vi "PS Control.vi"() -> ()   [LabVIEW 2025]
doc: "Author: Scott Hannahs <sth@magnet.fsu.edu>\n\nThis software is licensed for use under the “MIT License\"\nCopyright (c) 2025 Scott Hannahs, sth@sth@magnet.sthnet.net\n\nPermission is hereby granted, free of charge, to any person obtaining a copy of this software and associated documentation files (the \"Software\"), to deal in the Software without restriction, including without limitation the rights to use, copy, modify, merge, publish, distribute, sublicense, and/or sell copies of the Software, and to permit persons to whom the Software is furnished to do so, subject to the following conditions: The above copyright notice and this permission notice shall be included in all copies or substantial portions of the Software.\n\nTHE SOFTWARE IS PROVIDED \"AS IS\", WITHOUT WARRANTY OF ANY KIND, EXPRESS OR IMPLIED, INCLUDING BUT NOT LIMITED TO THE WARRANTIES OF MERCHANTABILITY, FITNESS FOR A PARTICULAR PURPOSE AND NONINFRINGEMENT. IN NO EVENT SHALL THE AUTHORS OR COPYRIGHT HOLDERS BE LIABLE FOR ANY CLAIM, DAMAGES OR OTHER LIABILITY, WHETHER IN AN ACTION OF CONTRACT, TORT OR OTHERWISE, ARISING FROM, OUT OF OR IN CONNECTION WITH THE SOFTWARE OR THE USE OR OTHER DEALINGS IN THE SOFTWARE."
panel:
  out "Power Supply State":T1(ring)
  out "Switch Heater":bool
  in  "stop":bool
  in  "Hold":bool
  in  "Ramp to Setpoint":bool
  out "Magnet Voltage":dbl format="%_3f"
  out "Field [T]":dbl format="%_6f"
  out "PS Response":string
  in  "IP Address":string
  in  "Slew Rate [T/min]":dbl format="%_6f"
  in  "Setpoint [T]":dbl format="%_6f"
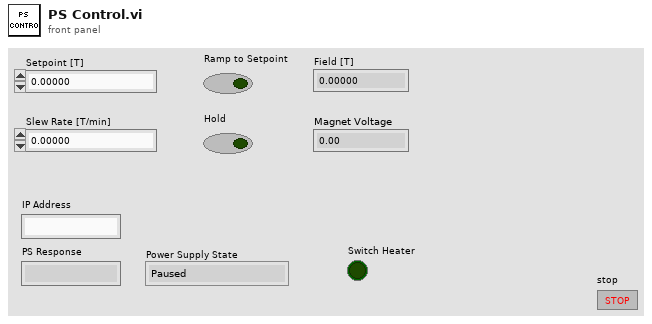
[diagram p1: front panel]
types:
  T1 = enum16{"Paused", "Ramping to Programmed Field", "QUENCH"}
  T2 = cluster{"Breakpts [A]":dbl[], "NormalRates [A/min]":dbl[], "TrainRates [A/min]":dbl[], "SwitchHtrCurrent [mA]":dbl, "SwitchWaitTime [s]":dbl, "FieldCurrentRatio [T/A]":dbl, "StabilitySetting [%]":dbl, "MaxNormalCurrent [A]":dbl, "Magnet ID":string, "LambdaRates [A/min]":dbl[], "MaxLambdaCurrent [A]":dbl}
  T3 = enum16{"Normal", "Train", "Lambda", "Train & Lambda"}
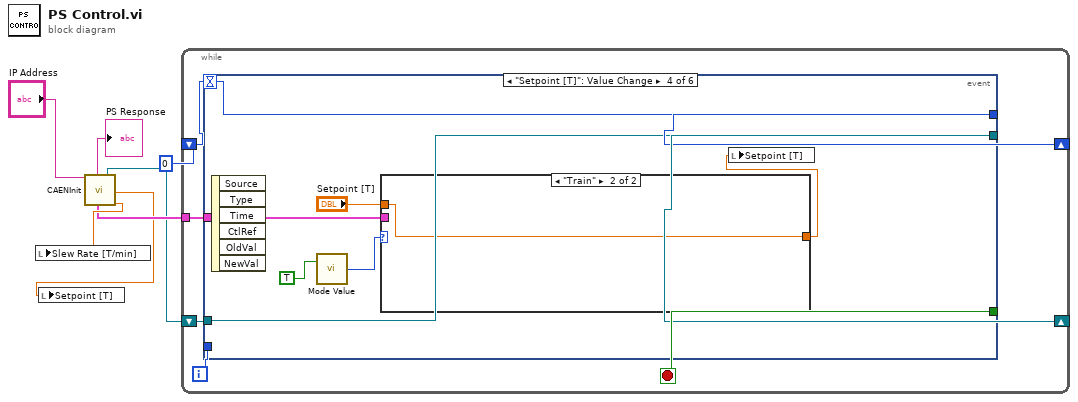
[diagram p0: block diagram]
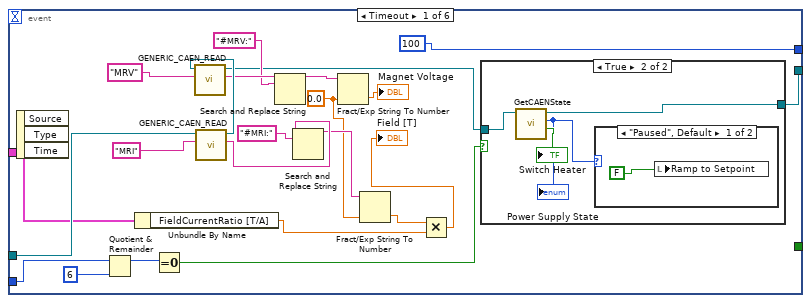
[diagram p2: hidden frame]
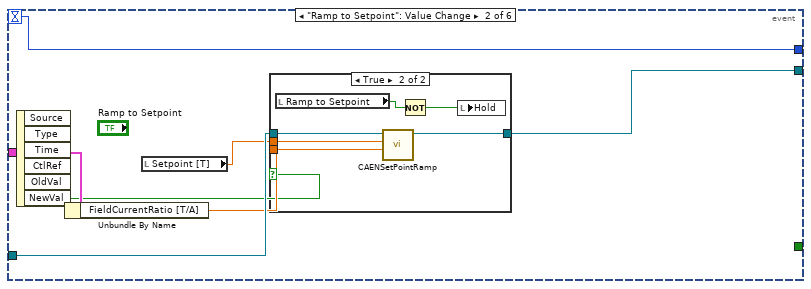
[diagram p5: hidden frame]
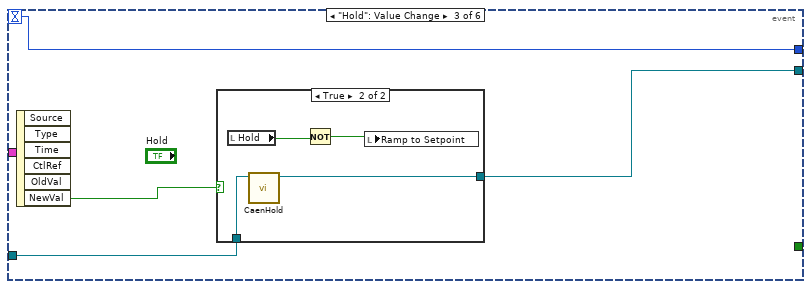
[diagram p7: hidden frame]
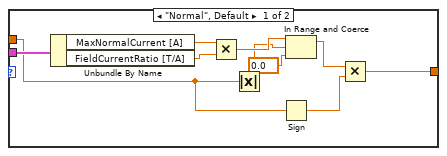
[diagram p9: hidden frame]
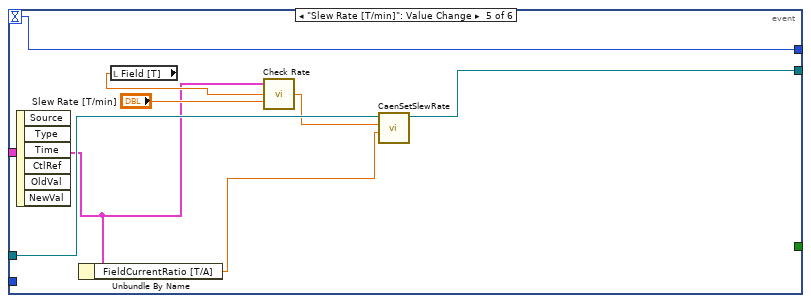
[diagram p10: hidden frame]
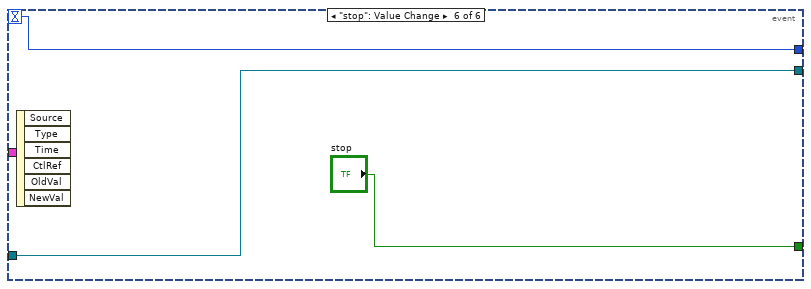
[diagram p11: hidden frame]
diagram:
  n1 = call "CAENInit.vi"("IP Address"="IP Address") -> ("Power Supply Response"=→"PS Response":string, "Output Cluster"=w4:T2, "Network Session Out"=w2:refnum<k5>, "Field Set Point"=w3:dbl, "Field Ramp Rate (T/min)"=w5:dbl)  [unwired: 8 in, 6 out]
  n2 = local write "Slew Rate [T/min]"(w5) -> ()
  n3 = local write "Setpoint [T]"(w3) -> ()
  n4 = while {
    tunnel: w4 -> [w13]
    shift-right: [w11] -> _
    shift-left: w2 -> [w12]
    shift-right: [w9] -> _
    shift-left: 0 -> [w10]
    i -> [w8]
    stop <- w14 stop-if-true
    n5 = event shown="[3] \"Setpoint [T]\": Value Change" {
      selector: _ -> [_ _ _ _ _ _]
      dyn-events: _ -> [_ _ _ _ _ _]
      timeout: w10 -> [_ w50 w61 w73 w92 w94]
      tunnel: [_ _ _ _ _ "stop"] -> w14
      tunnel: w12 -> [w35 w49 w60 w72 w91 w93]
      tunnel: w13 -> [w18 w47 _ w68 w86 _]
      tunnel: [w19 w45 w59 w72 w89 w93] -> w11
      tunnel: [100 w50 w61 w73 w92 w94] -> w9
      tunnel: w8 -> [w24 _ _ _ _ _]
      event Timeout {
        w26 = 0.0
        n6 = event-data() -> ()  [unwired: 1 in, 3 out]
        n7 = Quotient & Remainder(x=w24, y=6) -> (x-y*floor(x/y)=w22:i32)  [unwired: 1 out]
        n8 = Unbundle By Name(w18) -> ("FieldCurrentRatio [T/A]"=w17:dbl)
        n9 = Equal To 0?(x=w22) -> (x = 0?=w21:bool)
        n10 = call "GENERIC_CAEN_READ.vi"("String"="MRI", "Network Session"=w35) -> ("String 2"=w29:string, "Network Session Out"=w34:refnum<k5>)  [unwired: 7 in, 1 out]
        n11 = call "GENERIC_CAEN_READ.vi"("String"="MRV", "Network Session"=w34) -> ("String 2"=w33:string, "Network Session Out"=w20:refnum<k5>)  [unwired: 7 in, 1 out]
        n12 = Search and Replace String(input string=w33, search string="#MRV:") -> (result string=w31:string)  [unwired: 6 in, 3 out]
        n13 = Search and Replace String(input string=w29, search string="#MRI:") -> (result string=w27:string)  [unwired: 6 in, 3 out]
        n14 = Fract/Exp String To Number(string=w31, default (0 dbl)=w26) -> (number=→"Magnet Voltage":dbl)  [unwired: 2 in, 1 out]
        n15 = Fract/Exp String To Number(string=w27, default (0 dbl)=w26) -> (number=w16:dbl)  [unwired: 2 in, 1 out]
        n16 = Multiply(x=w16, y=w17) -> (x*y=→"Field [T]":dbl)
        n17 = case shown="True" w21 {
          tunnel: w20 -> [w38 w42]
          tunnel: [w38 w41] -> w19
          frame False {
          }
          frame True {
            n18 = call "GetCAENState.vi"("TCP Session"=w42) -> ("Switch Heater"=→"Switch Heater":bool, "Enum"=w39:T1, "TCP Session Out"=w41:refnum<k5>)  [unwired: 7 in, 1 out]
            "Power Supply State" <- w39
            n19 = case shown="\"Paused\", Default" w39 {
              frame "Paused", Default {
                n20 = local write "Ramp to Setpoint"(FALSE) -> ()
              }
              frame "Ramping to Programmed Field" {
              }
            }
          }
        }
      }
      event "Ramp to Setpoint": Value Change {
        n21 = event-data() -> ("NewVal"=w44:bool)  [unwired: 1 in, 5 out]
        n22 = Unbundle By Name(w47) -> ("FieldCurrentRatio [T/A]"=w46:dbl)
        n23 = local read "Setpoint [T]"() -> (w48:dbl)
        n24 = case shown="True" w44 {
          tunnel: w49 -> [w51 w57]
          tunnel: w48 -> [_ w56]
          tunnel: w46 -> [_ w55]
          tunnel: [w51 w54] -> w45
          frame False {
          }
          frame True {
            n25 = local read "Ramp to Setpoint"() -> (w53:bool)
            n26 = call "CAENSetPointRamp.vi"("Field/Current Ratio"=w55, "Setpoint [T]"=w56, "Network Session"=w57) -> ("Network Session Out"=w54:refnum<k5>)  [unwired: 6 in, 2 out]
            n27 = Not(x=w53) -> (.not. x?=w52:bool)
            n28 = local write "Hold"(w52) -> ()
          }
        }
      }
      event "Hold": Value Change {
        n29 = event-data() -> ("NewVal"=w58:bool)  [unwired: 1 in, 5 out]
        n30 = case shown="True" w58 {
          tunnel: w60 -> [w62 w66]
          tunnel: [w62 w65] -> w59
          frame False {
          }
          frame True {
            n31 = local read "Hold"() -> (w64:bool)
            n32 = call "CaenHold.vi"("Network Session"=w66) -> ("Network Session Out"=w65:refnum<k5>)  [unwired: 7 in, 3 out]
            n33 = Not(x=w64) -> (.not. x?=w63:bool)
            n34 = local write "Ramp to Setpoint"(w63) -> ()
          }
        }
      }
      event "Setpoint [T]": Value Change {
        n35 = event-data() -> ()  [unwired: 1 in, 6 out]
        n36 = call "Mode Value.vi"("Read/Write this vi"=TRUE) -> ("Mode Out"=w71:T3)  [unwired: 1 in]
        n37 = case shown="\"Train\"" w71 {
          tunnel: "Setpoint [T]" -> [w77 w84]
          tunnel: w68 -> [w83 _]
          tunnel: [w74 w84] -> w67
          frame "Normal", Default {
            n38 = Unbundle By Name(w83) -> ("MaxNormalCurrent [A]"=w82:dbl, "FieldCurrentRatio [T/A]"=w81:dbl)
            n39 = Multiply(x=w82, y=w81) -> (x*y=w80:dbl)
            n40 = Absolute Value(x=w77) -> (abs(x)=w78:dbl)
            n41 = Sign(1:w77) -> (0:w76:dbl)
            n42 = In Range and Coerce(upper limit=w80, x=w78, lower limit=0.0) -> (coerced(x)=w75:dbl)  [unwired: 1 out]
            n43 = Multiply(x=w75, y=w76) -> (x*y=w74:dbl)
          }
          frame "Train" {
          }
        }
        n44 = local write "Setpoint [T]"(w67) -> ()
      }
      event "Slew Rate [T/min]": Value Change {
        n45 = event-data() -> ()  [unwired: 1 in, 6 out]
        n46 = Unbundle By Name(w86) -> ("FieldCurrentRatio [T/A]"=w90:dbl)
        n47 = local read "Field [T]"() -> (w87:dbl)
        n48 = call "Check Rate.vi"("Rate"="Slew Rate [T/min]", "Field"=w87, "input cluster"=w86) -> ("Checked Rate"=w85:dbl)
        n49 = call "CaenSetSlewRate.vi"("Field Ratio"=w90, "Slew Rate [T/min]"=w85, "Network Session In"=w91) -> ("Network Session Out"=w89:refnum<k5>)  [unwired: 7 in, 1 out]
      }
      event "stop": Value Change {
        n50 = event-data() -> ()  [unwired: 1 in, 6 out]
      }
    }
  }
